vi "Get Set Speed.vi"(10 "Target Speed (Hz)":u32, 11 "Device Name":string="Basys2") -> (0 "Error Out":errorcluster, 3 "JTAG Speed (Hz)":u32, 7 "Actual JTAG Speed (Hz)":u32)   [LabVIEW 2011, in "LVH-Adept.lvlib"]
uses:
  <vilib>/LabVIEW Hacker/Adept/LVH-Adept.lvlib
  Private/DMGR/DMGR.lvlib
  Private/DJTG/DJTG.lvlib
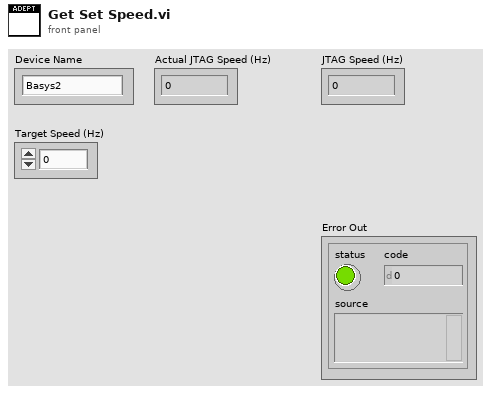
[diagram p1: front panel]
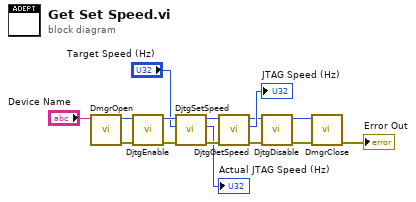
[diagram p0: block diagram]
diagram:
  n1 = call "DmgrOpen.vi"("Device Name"="Device Name") -> ("Error Out"=w11:errorcluster, "Device Handle"=w12:u32)  [unwired: 9 in]
  n2 = call "DjtgEnable.vi"("Error In"=w11, "Device Number"=w12) -> ("Error Out"=w6:errorcluster, "Device Number"=w5:u32)  [unwired: 8 in]
  n3 = call "DjtgSetSpeed.vi"("Error In"=w6, "Target Speed (Hz)"="Target Speed (Hz)", "Device Number"=w5) -> ("Error Out"=w3:errorcluster, "Actual JTAG Speed (Hz)"=→"Actual JTAG Speed (Hz)":u32, "Device Number"=w2:u32)  [unwired: 6 in]
  n4 = call "DjtgGetSpeed.vi"("Error In"=w3, "Device Number"=w2) -> ("Error Out"=w9:errorcluster, "JTAG Speed (Hz)"=→"JTAG Speed (Hz)":u32, "Device Number"=w10:u32)  [unwired: 7 in]
  n5 = call "DjtgDisable.vi"("Error In"=w9, "Device Number"=w10) -> ("Error Out"=w8:errorcluster, "Device Number"=w7:u32)  [unwired: 8 in]
  n6 = call "DmgrClose.vi"("Error In"=w8, "hif"=w7) -> ("Error Out"=→"Error Out":errorcluster)  [unwired: 9 in]
